vi "[subVI]_get_distance_data.vi"(8 "error in":errorcluster, 11 "COM in":refnum<visa-resource-name>) -> (0 "error out":errorcluster, 2 "S300 data":string, 3 "COM out":refnum<visa-resource-name>)   [LabVIEW 2013]
panel:
  # "Outputs"
  # "Inputs"
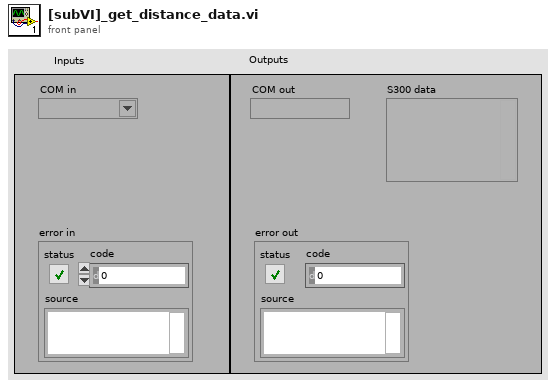
[diagram p1: front panel]
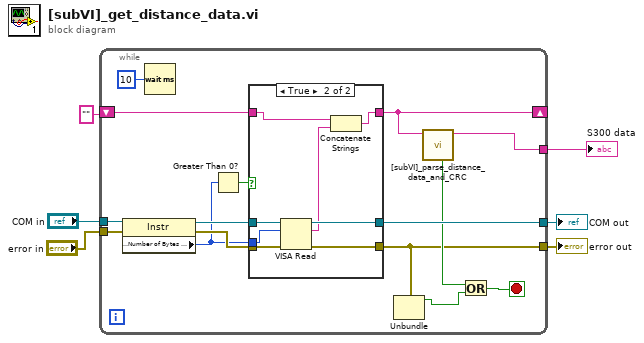
[diagram p0: block diagram]
diagram:
  n1 = while {
    tunnel: "COM in" -> [w21]
    tunnel: [w19] -> w4
    tunnel: [w8] -> w3
    tunnel: "error in" -> [w17]
    shift-right: [w11] -> _
    shift-left: "" -> [w14]
    tunnel: [w10] -> w5
    stop <- w13 stop-if-true
    n2 = property class="Instr"(reference=w21, error in=w17) -> (reference out=w20:refnum<visa-resource-name>, error out=w18:errorcluster, "Serial Settings:Number of Bytes at Serial Port"=w15:u32)
    n3 = Wait (ms)(milliseconds to wait=u32 10) -> ()  [unwired: 1 out]
    n4 = Greater Than 0?(x=w15) -> (x > 0?=w16:bool)
    n5 = case shown="True" w16 {
      tunnel: w20 -> [w24 w32]
      tunnel: [w24 w31] -> w19
      tunnel: w18 -> [w23 w30]
      tunnel: [w23 w29] -> w8
      tunnel: w15 -> [_ w28]
      tunnel: w14 -> [w22 w27]
      tunnel: [w22 w26] -> w11
      frame False {
      }
      frame True {
        n6 = VISA Read(VISA resource name=w32, byte count=w28, error in (no error)=w30) -> (VISA resource name out=w31:refnum<visa-resource-name>, read buffer=w25:string, error out=w29:errorcluster)  [unwired: 1 out]
        n7 = Concatenate Strings(w27, w25) -> (w26:string)
      }
    }
    n8 = Unbundle(w8) -> ("status"=w7:bool)  [unwired: 2 out]
    n9 = call "[subVI]_parse_distance_data_and_CRC.vi"("S300 data (input)"=w11) -> ("distance data and CRC"=w10:string, "Stop?"=w12:bool)  [unwired: 9 in]
    n10 = Or(x=w12, y=w7) -> (x .or. y?=w13:bool)
  }
  "S300 data" <- w5
  "COM out" <- w4
  "error out" <- w3
